vi "Resistor Band Colors Tester.vi"() -> ()   [LabVIEW 2018, in "Resistor Band Colors.lvlib"]
uses:
  Resistor Band Colors.lvlib
panel:
  out "R12":u8
  out "G12":u8
  out "B12":u8
  out "R11":u8
  out "G11":u8
  out "B11":u8
  out "R10":u8
  out "G10":u8
  out "B10":u8
  out "R9":u8
  out "G9":u8
  out "B9":u8
  out "R8":u8
  out "G8":u8
  out "B8":u8
  out "R7":u8
  out "G7":u8
  out "B7":u8
  out "R6":u8
  out "G6":u8
  out "B6":u8
  out "R5":u8
  out "G5":u8
  out "B5":u8
  out "R4":u8
  out "G4":u8
  out "B4":u8
  out "B3":u8
  out "G3":u8
  out "R3":u8
  out "B2":u8
  out "G2":u8
  out "R2":u8
  out "B1":u8
  out "G1":u8
  out "R1":u8
  out "Brown":u32(colorbox)
  out "Gold":u32(colorbox)
  out "Gray":u32(colorbox)
  out "Violet":u32(colorbox)
  out "Green":u32(colorbox)
  out "White":u32(colorbox)
  out "Orange":u32(colorbox)
  out "Red":u32(colorbox)
  out "Silver":u32(colorbox)
  out "Yellow":u32(colorbox)
  out "Blue":u32(colorbox)
  out "Black":u32(colorbox)
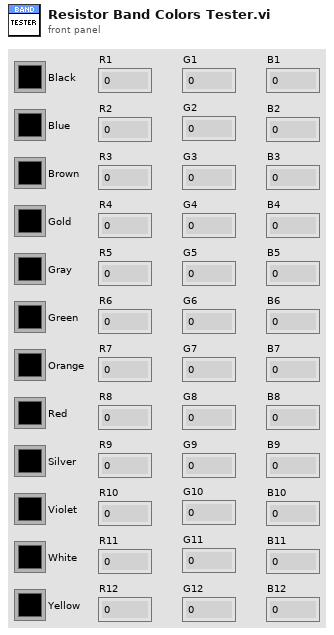
[diagram p1: front panel]
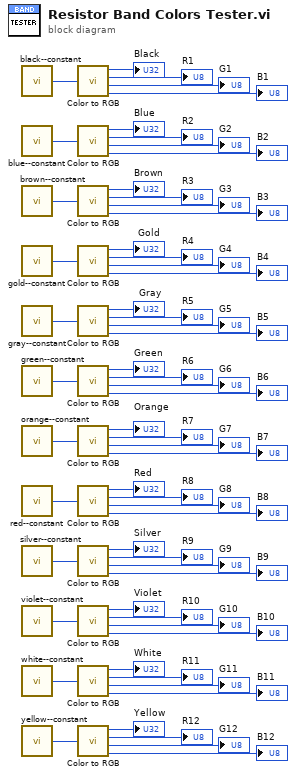
[diagram p0: block diagram]
diagram:
  n1 = call "black--constant.vi"() -> ("Black"=w59:u32)  [unwired: 5 in]
  n2 = call "blue--constant.vi"() -> ("Blue"=w55:u32)  [unwired: 5 in]
  n3 = call "brown--constant.vi"() -> ("Brown"=w50:u32)  [unwired: 5 in]
  n4 = call "gold--constant.vi"() -> ("Gold"=w45:u32)  [unwired: 5 in]
  n5 = call "gray--constant.vi"() -> ("Gray"=w44:u32)  [unwired: 5 in]
  n6 = call "green--constant.vi"() -> ("Green"=w43:u32)  [unwired: 5 in]
  n7 = call "orange--constant.vi"() -> ("Orange"=w38:u32)  [unwired: 5 in]
  n8 = call "red--constant.vi"() -> ("Red"=w37:u32)  [unwired: 5 in]
  n9 = call "silver--constant.vi"() -> ("Silver"=w35:u32)  [unwired: 5 in]
  n10 = call "violet--constant.vi"() -> ("Violet"=w33:u32)  [unwired: 5 in]
  n11 = call "white--constant.vi"() -> ("White"=w32:u32)  [unwired: 5 in]
  n12 = call "yellow--constant.vi"() -> ("Yellow"=w31:u32)  [unwired: 5 in]
  n13 = call <vilib>:"Color to RGB.vi"("Color"=w59) -> ("Resolved Color"=→"Black":u32, "R"=→"R1":u8, "G"=→"G1":u8, "B"=→"B1":u8)
  n14 = call <vilib>:"Color to RGB.vi"("Color"=w55) -> ("Resolved Color"=→"Blue":u32, "R"=→"R2":u8, "G"=→"G2":u8, "B"=→"B2":u8)
  n15 = call <vilib>:"Color to RGB.vi"("Color"=w50) -> ("Resolved Color"=→"Brown":u32, "R"=→"R3":u8, "G"=→"G3":u8, "B"=→"B3":u8)
  n16 = call <vilib>:"Color to RGB.vi"("Color"=w45) -> ("Resolved Color"=→"Gold":u32, "R"=→"R4":u8, "G"=→"G4":u8, "B"=→"B4":u8)
  n17 = call <vilib>:"Color to RGB.vi"("Color"=w44) -> ("Resolved Color"=→"Gray":u32, "R"=→"R5":u8, "G"=→"G5":u8, "B"=→"B5":u8)
  n18 = call <vilib>:"Color to RGB.vi"("Color"=w43) -> ("Resolved Color"=→"Green":u32, "R"=→"R6":u8, "G"=→"G6":u8, "B"=→"B6":u8)
  n19 = call <vilib>:"Color to RGB.vi"("Color"=w38) -> ("Resolved Color"=→"Orange":u32, "R"=→"R7":u8, "G"=→"G7":u8, "B"=→"B7":u8)
  n20 = call <vilib>:"Color to RGB.vi"("Color"=w37) -> ("Resolved Color"=→"Red":u32, "R"=→"R8":u8, "G"=→"G8":u8, "B"=→"B8":u8)
  n21 = call <vilib>:"Color to RGB.vi"("Color"=w35) -> ("Resolved Color"=→"Silver":u32, "R"=→"R9":u8, "G"=→"G9":u8, "B"=→"B9":u8)
  n22 = call <vilib>:"Color to RGB.vi"("Color"=w33) -> ("Resolved Color"=→"Violet":u32, "R"=→"R10":u8, "G"=→"G10":u8, "B"=→"B10":u8)
  n23 = call <vilib>:"Color to RGB.vi"("Color"=w32) -> ("Resolved Color"=→"White":u32, "R"=→"R11":u8, "G"=→"G11":u8, "B"=→"B11":u8)
  n24 = call <vilib>:"Color to RGB.vi"("Color"=w31) -> ("Resolved Color"=→"Yellow":u32, "R"=→"R12":u8, "G"=→"G12":u8, "B"=→"B12":u8)
